vi "Reporting_ini.vi"(2 "Configuration cluster":T1, 3 "address repoting":path) -> (1 "Reporting":string)   [LabVIEW 2015]
panel:
  out "error out":errorcluster
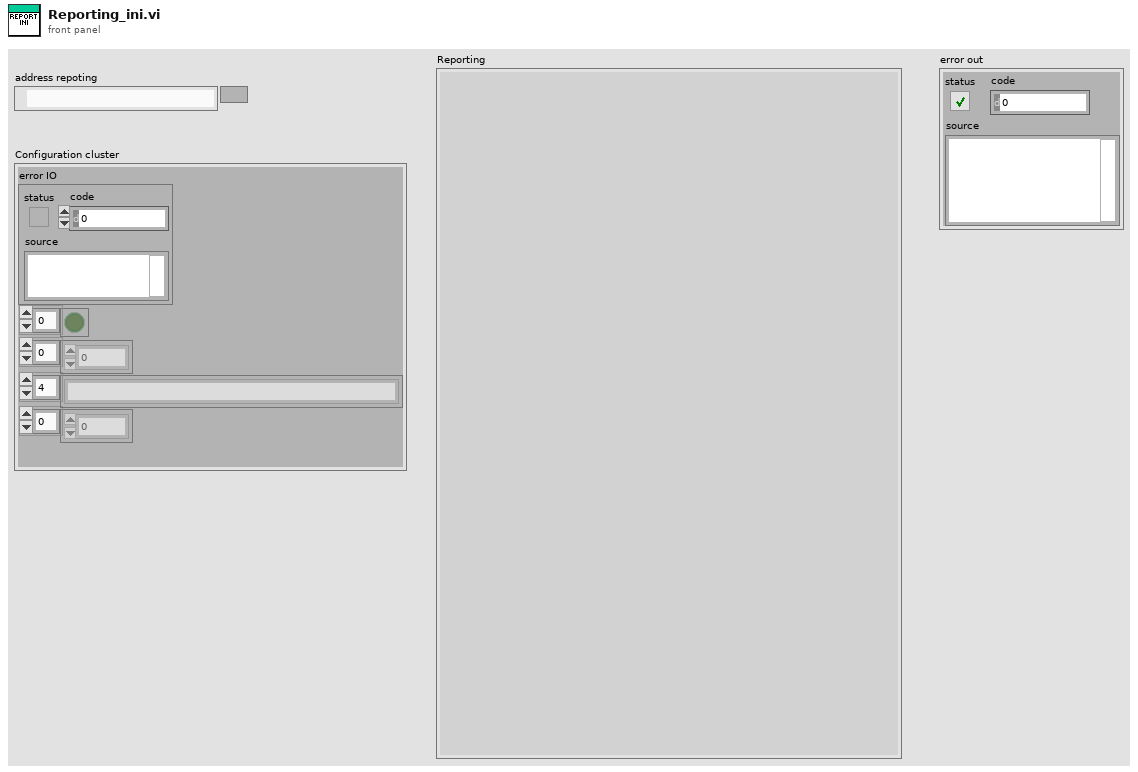
[diagram p1: front panel]
types:
  T1 = cluster{"error IO":errorcluster, bool[], u32[], string[], dbl[]}
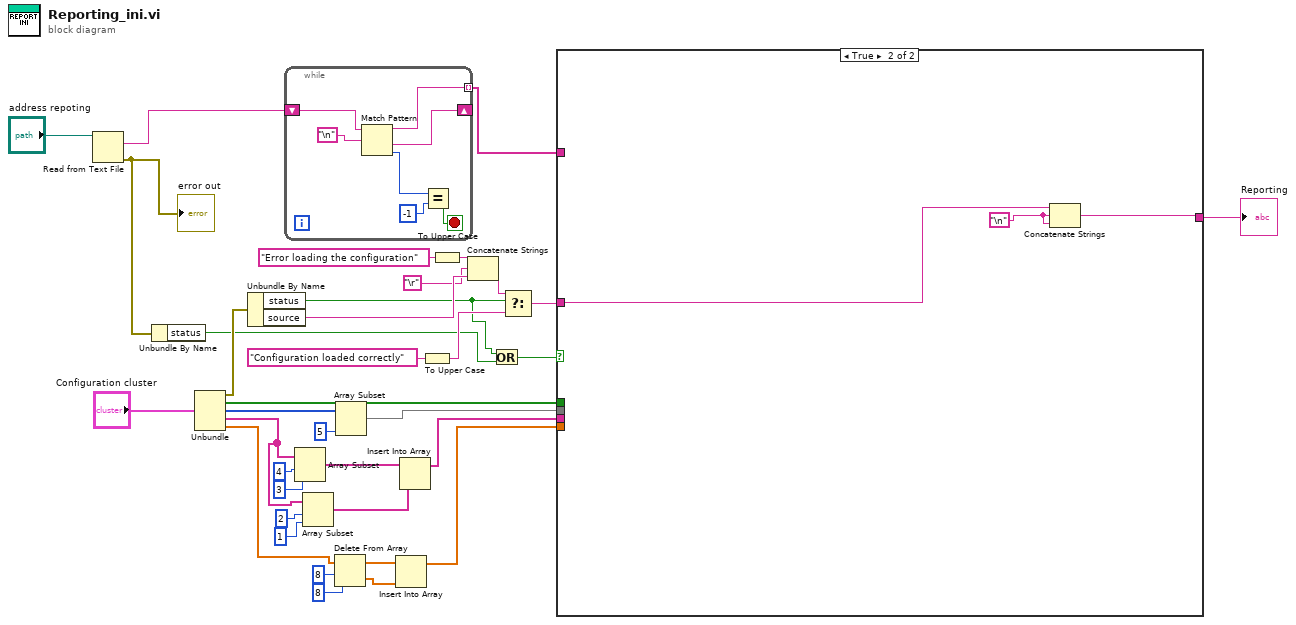
[diagram p0: block diagram]
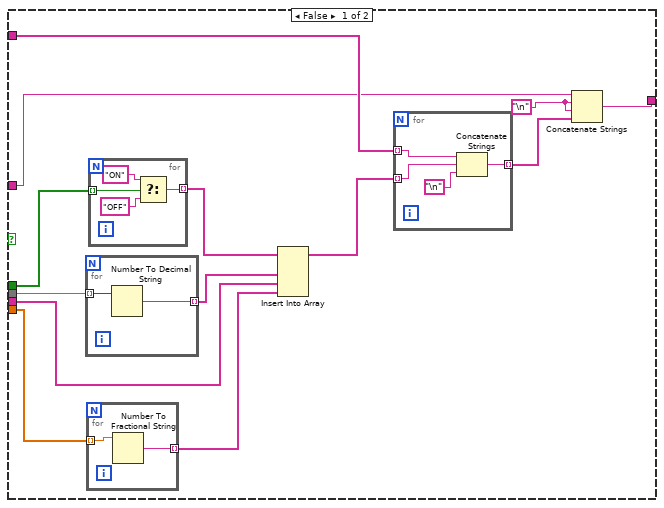
[diagram p2: hidden frame]
diagram:
  n1 = Read from Text File(file (use dialog)="address repoting") -> (text=w36:string, error out=w4:errorcluster)  [unwired: 3 in, 2 out]
  "error out" <- w4
  n2 = Unbundle By Name(w4) -> ("status"=w1:bool)
  n3 = Unbundle("Configuration cluster") -> ("error IO"=w31:errorcluster, w28:bool[], w25:u32[], w6:string[], w18:dbl[])
  n4 = Unbundle By Name(w31) -> ("status"=w3:bool, "source"=w33:string)
  n5 = while {
    tunnel: [w40] -> w27 mode=indexing
    shift-right: [w37] -> _
    shift-left: w36 -> [w38]
    stop <- w43 stop-if-true
    n6 = Match Pattern(string=w38, regular expression="\n") -> (before substring=w40:string, after substring=w37:string, offset past match=w41:i32)  [unwired: 1 in, 1 out]
    n7 = Equal?(x=w41, y=-1) -> (x = y?=w43:bool)
  }
  n8 = Array Subset(array=w6, index=4 ("length"), length=3 ("index")) -> (w5:string[])
  n9 = Array Subset(array=w6, index=2 ("length"), length=1) -> (w7:string[])
  n10 = Delete From Array(array=w18, length=8, index=8) -> (deleted portion=w16:dbl[], array with subset deleted=w17:dbl[])
  n11 = Array Subset(array=w25, length=5) -> (w23:u32[])  [unwired: 1 in]
  n12 = Insert Into Array(array=w17, new element=w16) -> (w15:dbl[])  [unwired: 1 in]
  n13 = Insert Into Array(array=w5, new element=w7) -> (w8:string[])  [unwired: 1 in]
  n14 = To Upper Case(1:"Configuration loaded correctly") -> (0:w13:string)
  n15 = To Upper Case(1:"Error loading the configuration") -> (0:w11:string)
  n16 = Concatenate Strings(w11, "\r", w33) -> (w26:string)
  n17 = Or(x=w3, y=w1) -> (x .or. y?=w2:bool)
  n18 = Select(t=w26, s=w3, f=w13) -> (s? t:f=w30:string)
  n19 = case shown="True" w2 {
    tunnel: w30 -> [w47 w70]
    tunnel: [w46 w69] -> w29
    tunnel: w28 -> [w56 _]
    tunnel: w23 -> [w55 _]
    tunnel: w8 -> [w51 _]
    tunnel: w15 -> [w54 _]
    tunnel: w27 -> [w49 _]
    frame False {
      w44 = "\n"
      n20 = for {
        tunnel: w55 -> [w64] mode=indexing
        tunnel: [w63] -> w52 mode=indexing
        n21 = Number To Decimal String(number=w64) -> (decimal integer string=w63:string)  [unwired: 1 in]
      }
      n22 = for {
        tunnel: w54 -> [w62] mode=indexing
        tunnel: [w61] -> w50 mode=indexing
        n23 = Number To Fractional String(number=w62) -> (F-format string=w61:string)  [unwired: 3 in]
      }
      n24 = for {
        tunnel: w56 -> [w68] mode=indexing
        tunnel: [w65] -> w53 mode=indexing
        n25 = Select(t="ON", s=w68, f="OFF") -> (s? t:f=w65:string)
      }
      n26 = Insert Into Array(array=w53, new element #1=w52, new element #2=w51, new element #3=w50) -> (w48:string[])  [unwired: 1 in]
      n27 = for {
        tunnel: w49 -> [w60] mode=indexing
        tunnel: w48 -> [w59] mode=indexing
        tunnel: [w57] -> w45 mode=indexing
        n28 = Concatenate Strings(w60, w59, "\n") -> (w57:string)
      }
      n29 = Concatenate Strings(w47, w44, w44, w45) -> (w46:string)
    }
    frame True {
      w71 = "\n"
      n30 = Concatenate Strings(w70, w71, w71) -> (w69:string)
    }
  }
  "Reporting" <- w29
